vi "Teleop.vi"(10 "Match Info":T1={"Autonomous Elapsed Seconds"=0.0, "TeleOp Elapsed Seconds"=0.0, "Disabled Elapsed Seconds"=0.0, "Visited Autonomous"=FALSE, "Visited TeleOp"=FALSE, "Visited Disabled"=FALSE, "Autonomous Settings"={"Autonomous Style"=enum."Independent", "VI Refnum"=refnum}}, 11 "Call Context":T2) -> ()   [LabVIEW 2019]
doc: "This VI is called for each enabled TeleOp packet received from the DS. It is typically used to read from joysticks and other inputs and update I/O or setpoints for timed control loops. It should complete and return within 20 milliseconds or risk missing DS packets."
uses:
  Support Code/Controller Buttons.ctl
  <vilib>/Rock Robotics/WPI/DriverStation/WPI_DriverStationMatch Info.ctl
  <vilib>/Rock Robotics/WPI/DriverStation/WPI_DriverStationDerivedRobotMode.ctl
panel:
  in  "Hood Position":dbl(slide) scale=0.0..100.0
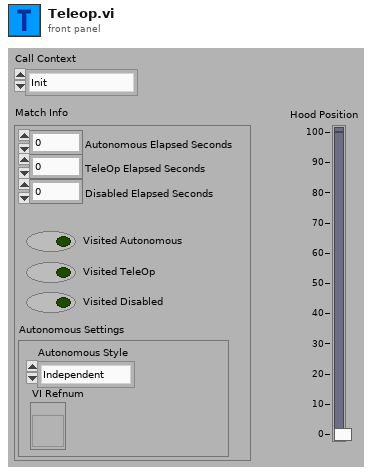
[diagram p1: front panel]
types:
  T1 = typedef "WPI_DriverStationMatch Info.ctl" = cluster{"Autonomous Elapsed Seconds":dbl, "TeleOp Elapsed Seconds":dbl, "Disabled Elapsed Seconds":dbl, "Visited Autonomous":bool, "Visited TeleOp":bool, "Visited Disabled":bool, "Autonomous Settings":cluster{"Autonomous Style":enum16{"Iterative", "Independent"}, "VI Refnum":refnum<vi>}}
  T2 = typedef "WPI_DriverStationDerivedRobotMode.ctl" = enum16{"Init", "Execute", "Stop"}
  T3 = typedef "Controller Buttons.ctl" = enum32{"A", "B", "X", "Y", "Left Bumper", "Right Bumper", "Select", "Start", "Left Joystick Button", "Right Joystick Button"}
  T4 = typedef "WPI_JoystickDevRef.ctl" = cluster{"Device":T5}
  T5 = typedef "WPI_JoystickDeviceEnum.ctl" = enum16{"USB 0", "USB 1", "USB 2", "USB 3", "USB 4", "USB 5"}
  T6 = typedef "Command Status Info.ctl" = cluster{"Name":string, "Status":T7, "notifier out":T8}
  T7 = typedef "Completion Status.ctl" = enum16{"Successful", "Aborted", "Incomplete"}
  T8 = typedef "Completion Notifier.ctl" = refnum<notifier>
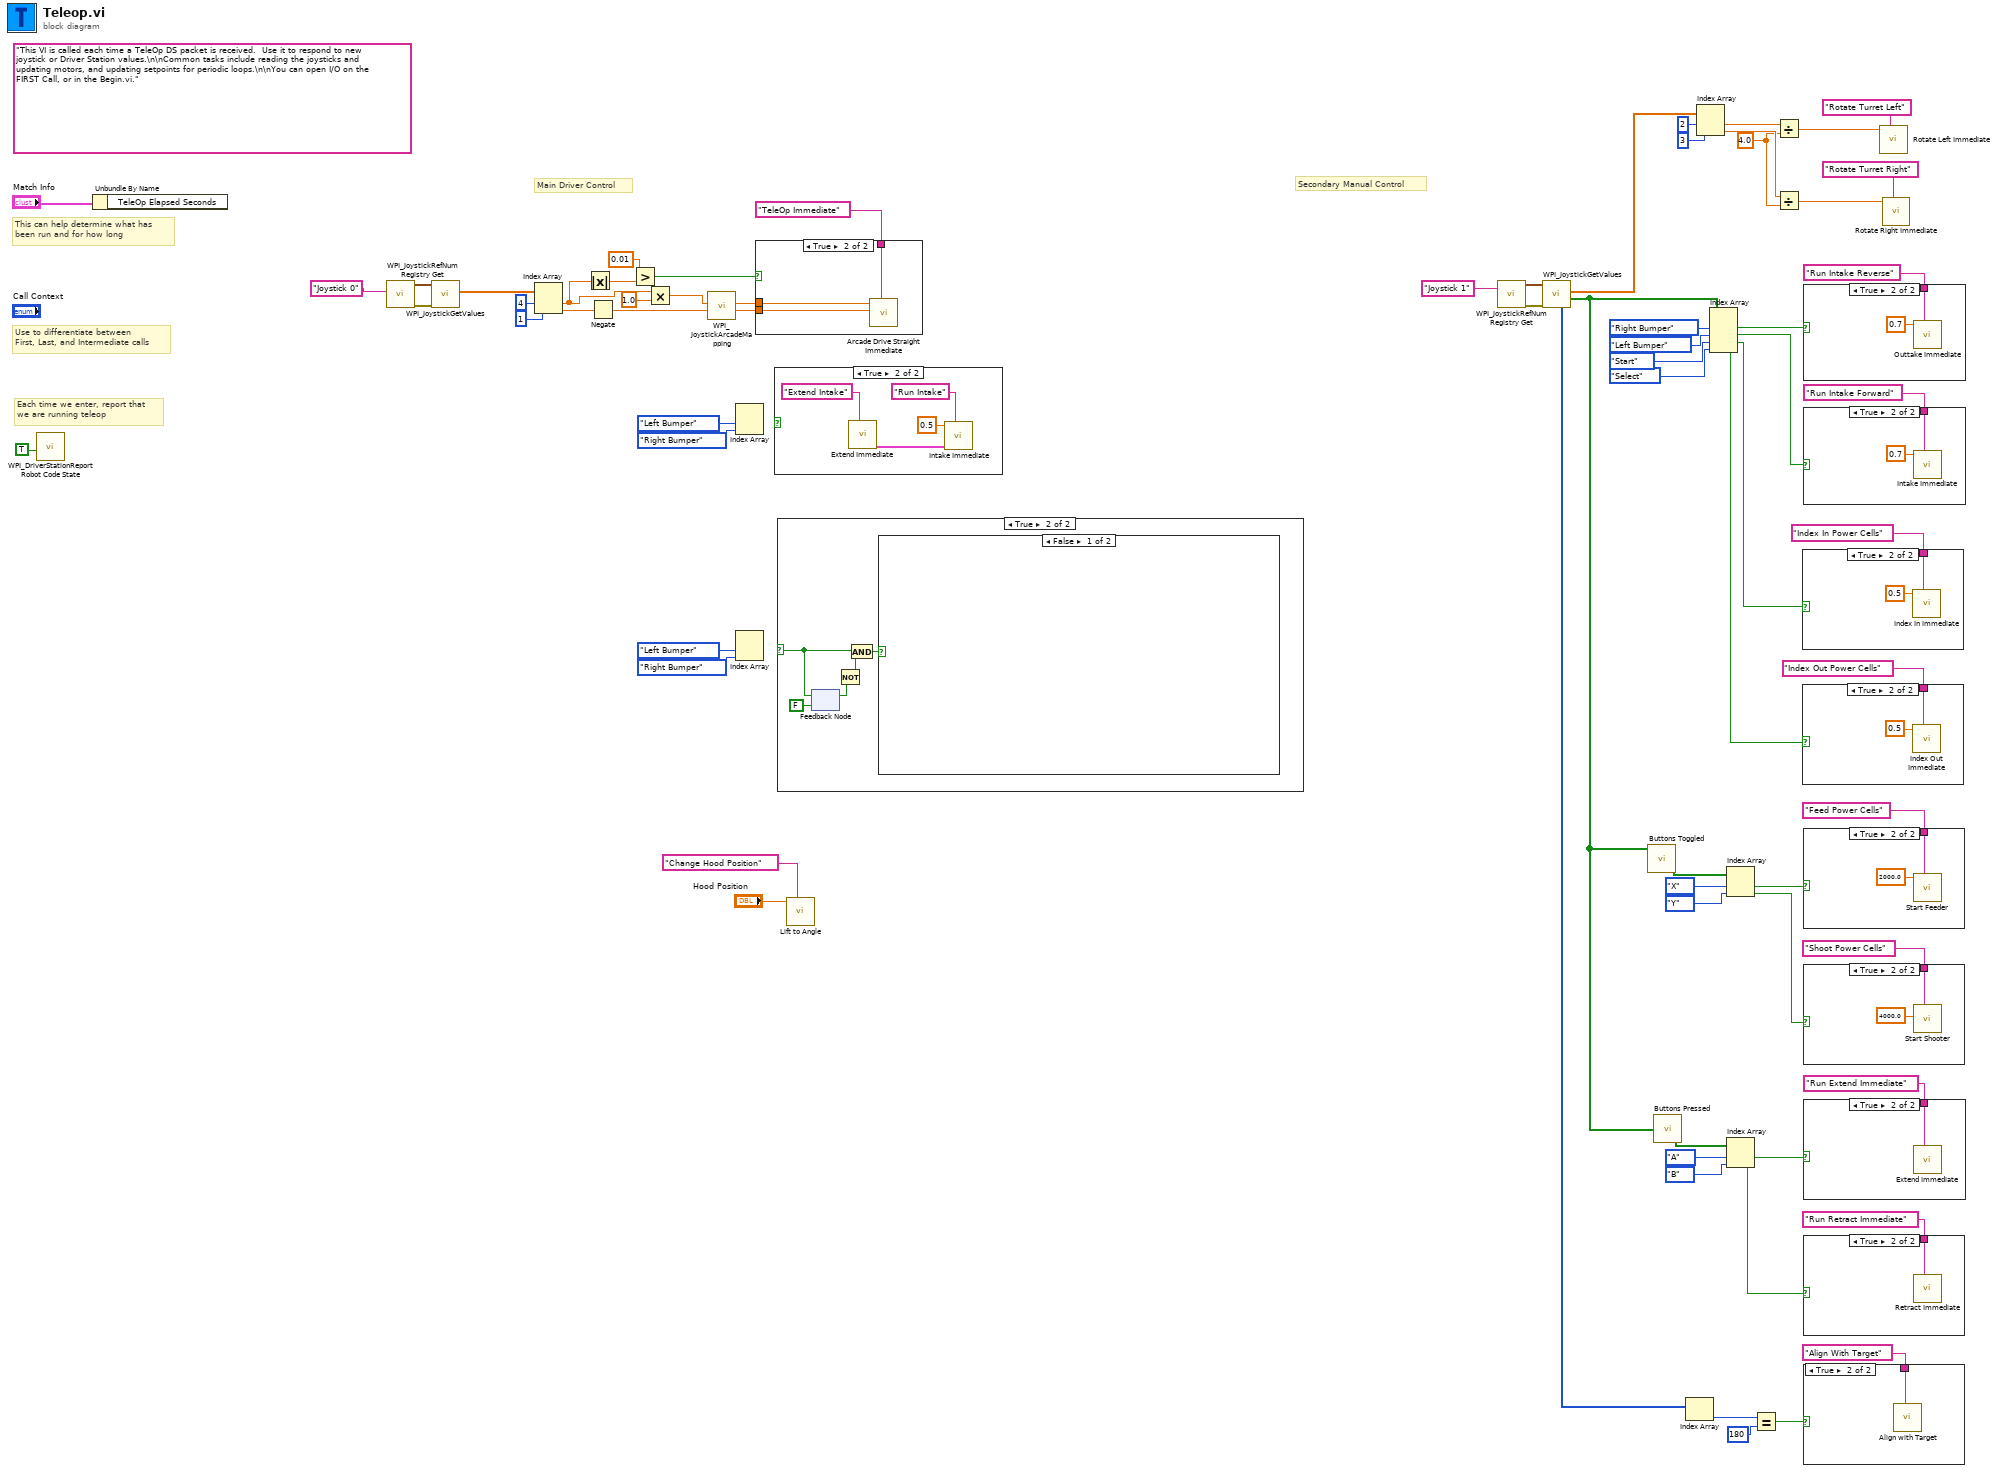
[diagram p0: block diagram]
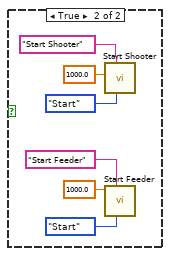
[diagram p3: hidden frame]
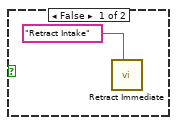
[diagram p4: hidden frame]
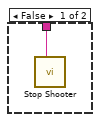
[diagram p8: hidden frame]
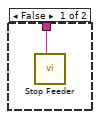
[diagram p9: hidden frame]
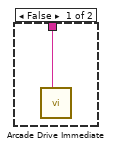
[diagram p14: hidden frame]
diagram:
  w13 = 4.0 ("y")
  (unwired) "This VI is called each time a TeleOp DS packet is received.  Use it to respond to new joystick or Driver Station values.\n\nCommon tasks include reading the joysticks and updating motors, and updating setpoints for periodic loops.\n\nYou can open I/O on the FIRST Call, or in the Begin.vi."
  # "Secondary Manual Control"
  # "Main Driver Control"
  # "Each time we enter, report that\nwe are running teleop"
  # "Use to differentiate between\nFirst, Last, and Intermediate calls"
  # "This can help determine what has\nbeen run and for how long"
  n1 = call <vilib>:"WPI_DriverStationReport Robot Code State.vi"("TeleOp"=TRUE ("Autonomous")) -> ()  [unwired: 10 in, 1 out]
  n2 = Unbundle By Name("Match Info") -> ()  [unwired: 1 out]
  n3 = call <vilib>:"WPI_JoystickRefNum Registry Get.vi"("refnum name"="Joystick 0") -> ("error out"=w53:errorcluster, "JoystickDevRef"=w67:T4)  [unwired: 1 in, 8 out]
  n4 = call <vilib>:"WPI_JoystickGetValues.vi"("error in (no error)"=w53, "JoystickDevRef"=w67) -> ("Axes"=w66:dbl[])  [unwired: 5 in, 4 out]
  n5 = Index Array(array=w66, index #1=4 ("index"), index #2=1 ("index")) -> (element #1=w10:dbl, element #2=w61:dbl)
  n6 = Absolute Value(x=w10) -> (abs(x)=w64:dbl)
  n7 = Negate(x=w61) -> (-x=w8:dbl)
  n8 = Greater?(x=0.01, y=w64) -> (0:w62:bool)
  n9 = Multiply(x=w10, y=1.0) -> (x*y=w7:dbl)
  n10 = call <vilib>:"WPI_JoystickArcadeMapping.vi"("Y axis value"=w8, "X axis value"=w7) -> ("Right Motor Value"=w5:dbl, "Left Motor Value"=w6:dbl)  [unwired: 8 in]
  n11 = Index Array(index #1=Controller_Buttons."Left Bumper" ("Controller Buttons"), index #2=Controller_Buttons."Right Bumper" ("Controller Buttons")) -> ()  [unwired: 1 in, 2 out]
  n12 = Index Array(index #1=Controller_Buttons."Left Bumper" ("Controller Buttons"), index #2=Controller_Buttons."Right Bumper" ("Controller Buttons")) -> ()  [unwired: 1 in, 2 out]
  n13 = case shown="True" w62 {
    tunnel: "TeleOp Immediate" ("Description") -> [w71 w74]
    tunnel: w6 -> [_ w73]
    tunnel: w5 -> [_ w72]
    frame False {
      n14 = call "Arcade Drive Immediate.vi"("Description"=w71) -> ()  [unwired: 10 in, 1 out]
    }
    frame True {
      n15 = call "Arcade Drive Straight Immediate.vi"("Description"=w74, "Right Setpoint"=w72, "Left Setpoint"=w73) -> ()  [unwired: 9 in]
    }
  }
  n16 = case shown="True" {
    selector: _ -> [_ _]
    frame False {
      n17 = call "Retract Immediate.vi"("Description"="Retract Intake") -> ()  [unwired: 10 in, 1 out]
    }
    frame True {
      n18 = call "Extend Immediate.vi"("Description"="Extend Intake") -> ("Command Info Out"=w78:T6)  [unwired: 10 in]
      n19 = call "Intake Immediate.vi"("Description"="Run Intake", "Command Info In"=w78, "Power"=0.5) -> ()  [unwired: 8 in, 1 out]
    }
  }
  n20 = case shown="True" {
    selector: _ -> [_ w82]
    frame False {
    }
    frame True {
      n21 = feedback-in #1(w82) -> ()
      n22 = feedback #1(FALSE) -> (w80:bool)
      n23 = Not(x=w80) -> (.not. x?=w81:bool)
      n24 = And(x=w82, y=w81) -> (x .and. y?=w83:bool)
      n25 = case shown="False" w83 {
        frame False {
        }
        frame True {
          n26 = call "Start Shooter.vi"("Synchronization"=enum16{"Start", "Wait"}."Start", "Description"="Start Shooter", "Velocity Setpoint (RPM)"=1000.0 ("Velocity")) -> ()  [unwired: 8 in, 1 out]
          n27 = call "Start Feeder.vi"("Synchronization"=enum16{"Start", "Wait"}."Start", "Description"="Start Feeder", "Velocity"=1000.0) -> ()  [unwired: 8 in, 1 out]
        }
      }
    }
  }
  n28 = call "Lift to Angle.vi"("Description"="Change Hood Position", "Angle"="Hood Position") -> ()  [unwired: 9 in, 1 out]
  n29 = call <vilib>:"WPI_JoystickRefNum Registry Get.vi"("refnum name"="Joystick 1") -> ("error out"=w54:errorcluster, "JoystickDevRef"=w55:T4)  [unwired: 1 in, 8 out]
  n30 = call <vilib>:"WPI_JoystickGetValues.vi"("error in (no error)"=w54, "JoystickDevRef"=w55) -> ("Buttons"=w42:bool[], "Axes"=w22:dbl[], "POVs"=w29:i16[])  [unwired: 5 in, 2 out]
  n31 = call "Buttons Toggled.vi"("Buttons"=w42) -> ("Buttons Toggled"=w48:bool[])  [unwired: 10 in]
  n32 = call "Buttons Pressed.vi"("Button Values"=w42) -> ("Button Presses"=w41:bool[])
  n33 = Index Array(array=w29) -> (element=w27:i16)  [unwired: 1 in]
  n34 = Index Array(array=w22, index #1=2 ("index"), index #2=3 ("index")) -> (element #1=w15:dbl, element #2=w14:dbl)
  n35 = Index Array(array=w42, index #1=Controller_Buttons."Right Bumper" ("Controller Buttons"), index #2=Controller_Buttons."Left Bumper" ("Controller Buttons"), index #3=Controller_Buttons."Start" ("Controller Buttons"), index #4=Controller_Buttons."Select" ("Controller Buttons")) -> (element #1=w60:bool, element #2=w59:bool, element #3=w35:bool, element #4=w33:bool)
  n36 = Index Array(array=w48, index #1=Controller_Buttons."X" ("Controller Buttons"), index #2=Controller_Buttons."Y" ("Controller Buttons")) -> (element #1=w47:bool, element #2=w46:bool)
  n37 = Index Array(array=w41, index #1=Controller_Buttons."A" ("Controller Buttons"), index #2=Controller_Buttons."B" ("Controller Buttons")) -> (element #1=w38:bool, element #2=w37:bool)
  n38 = Equal?(x=w27, y=i16 180) -> (x = y?=w26:bool)
  n39 = Divide(x=w15, y=w13) -> (x/y=w16:dbl)
  n40 = Divide(x=w14, y=w13) -> (x/y=w17:dbl)
  n41 = case shown="True" w35 {
    tunnel: "Index In Power Cells" ("Description") -> [_ w92]
    frame False {
    }
    frame True {
      n42 = call "Index In Immediate.vi"("Description"=w92, "Power"=0.5) -> ()  [unwired: 9 in, 1 out]
    }
  }
  n43 = case shown="True" w33 {
    tunnel: "Index Out Power Cells" ("Description") -> [_ w94]
    frame False {
    }
    frame True {
      n44 = call "Index Out Immediate.vi"("Description"=w94, "Power"=0.5) -> ()  [unwired: 9 in, 1 out]
    }
  }
  n45 = case shown="True" w60 {
    tunnel: "Run Intake Reverse" ("Description") -> [_ w95]
    frame False {
    }
    frame True {
      n46 = call "Outtake Immediate.vi"("Description"=w95, "Power"=0.7) -> ()  [unwired: 9 in, 1 out]
    }
  }
  n47 = case shown="True" w59 {
    tunnel: "Run Intake Forward" ("Description") -> [_ w97]
    frame False {
    }
    frame True {
      n48 = call "Intake Immediate.vi"("Description"=w97, "Power"=0.7) -> ()  [unwired: 9 in, 1 out]
    }
  }
  n49 = case shown="True" w47 {
    tunnel: "Feed Power Cells" ("Description") -> [w99 w101]
    frame False {
      n50 = call "Stop Feeder.vi"("Description"=w99) -> ()  [unwired: 10 in, 1 out]
    }
    frame True {
      n51 = call "Start Feeder.vi"("Description"=w101, "Velocity"=2000.0) -> ()  [unwired: 9 in, 1 out]
    }
  }
  n52 = case shown="True" w46 {
    tunnel: "Shoot Power Cells" ("Description") -> [w102 w104]
    frame False {
      n53 = call "Stop Shooter.vi"("Description"=w102) -> ()  [unwired: 10 in, 1 out]
    }
    frame True {
      n54 = call "Start Shooter.vi"("Description"=w104, "Velocity Setpoint (RPM)"=4000.0) -> ()  [unwired: 9 in, 1 out]
    }
  }
  n55 = case shown="True" w38 {
    tunnel: "Run Extend Immediate" ("Description") -> [_ w105]
    frame False {
    }
    frame True {
      n56 = call "Extend Immediate.vi"("Description"=w105) -> ()  [unwired: 10 in, 1 out]
    }
  }
  n57 = case shown="True" w37 {
    tunnel: "Run Retract Immediate" ("Description") -> [_ w106]
    frame False {
    }
    frame True {
      n58 = call "Retract Immediate.vi"("Description"=w106) -> ()  [unwired: 10 in, 1 out]
    }
  }
  n59 = case shown="True" w26 {
    tunnel: "Align With Target" ("Description") -> [_ w107]
    frame False {
    }
    frame True {
      n60 = call "Align with Target.vi"("Description"=w107) -> ()  [unwired: 10 in, 1 out]
    }
  }
  n61 = call "Rotate Left Immediate.vi"("Description"="Rotate Turret Left", "Power Setpoint"=w16) -> ()  [unwired: 9 in, 1 out]
  n62 = call "Rotate Right Immediate.vi"("Description"="Rotate Turret Right", "Setpoint"=w17) -> ()  [unwired: 9 in, 1 out]
